vi "Sum of 3 Gaussians with offset fit.vi"() -> ()   [LabVIEW 2023]
doc: "Demonstrates fitting data to a model that is the sum of three Gaussian curves and an offset."
uses:
  <vilib>/Analysis/1siggen.llb/Ramp Pattern by Samples.vi
  <vilib>/gmath/NumericalOptimization/Nonlinear Curve Fit LM.vi
  <vilib>/gmath/NI_Gmath.lvlib
  <vilib>/Analysis/NI_AALBase.lvlib
  <vilib>/Analysis/NI_AAL_SigProc.lvlib
panel:
  out "Sum of 3 Gaussians":T1(graph)
  out "Number of function calls":i32
  out "Residue":dbl
  out "DC offset fit":dbl
  out "Gauss 3 fit":cluster{"a":dbl, "m":dbl, "sigma":dbl}
  out "Gauss 2 fit":cluster{"a":dbl, "m":dbl, "sigma":dbl}
  out "Gauss 1 fit":cluster{"a":dbl, "m":dbl, "sigma":dbl}
  in  "DC offset":dbl=4.0
  in  "Gauss 3":cluster{"a":dbl, "m":dbl, "sigma":dbl}={"a"=3.0, "m"=0.3, "sigma"=0.03}
  in  "Gauss 2":cluster{"a":dbl, "m":dbl, "sigma":dbl}={"a"=2.0, "m"=0.2, "sigma"=0.02}
  in  "Gauss 1":cluster{"a":dbl, "m":dbl, "sigma":dbl}={"a"=1.0, "m"=0.1, "sigma"=0.01}
  in  "Noise sigma":dbl(slide)=0.050505050505050504 scale=0.0..0.1
  # "Overview: Demonstrates fitting data to a model that is the sum of three Gaussian curves and an offset.\nRequirements: LabVIEW Full Development System\nInstructions:\n1.  Run the VI.\n2.  Notice the fit, which is mostly good.  Sometimes the smallest peak is missed due to the starting set of parameters for the fit.\n3.  Change the Gaussian parameters (DC offset, Gauss 1, Gauss 2, and Gauss 3) or Noise sigma and run the VI again."
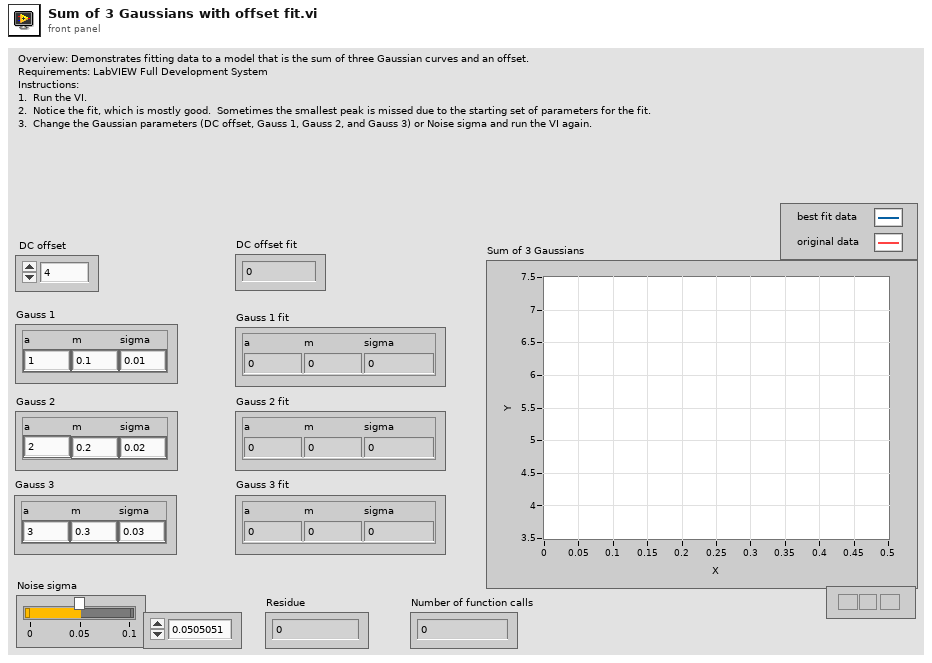
[diagram p1: front panel]
types:
  T1 = cluster{"Ramp Pattern":dbl[], "best nonlinear fit":dbl[]}[]
  T2 = cluster{"Ramp Pattern":dbl[], "best nonlinear fit":dbl[]}
  T3 = cluster{"Numeric":dbl, "Numeric":dbl, "Numeric":dbl}
  T4 = cluster{"Numeric":dbl, "Numeric":dbl, "Numeric":dbl}[]
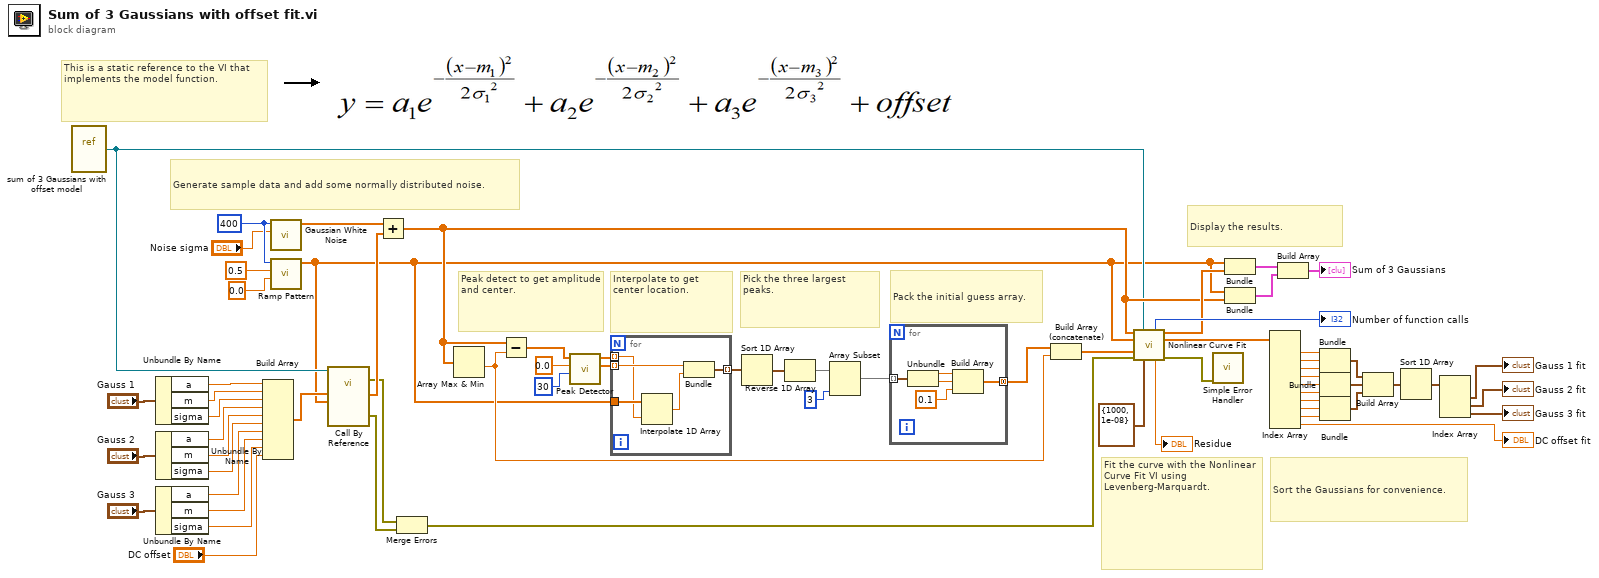
[diagram p0: block diagram]
diagram:
  w53 = 400 ("samples")
  # "Pack the initial guess array."
  # "Pick the three largest peaks."
  # "Peak detect to get amplitude and center."
  # "Sort the Gaussians for convenience."
  # "Generate sample data and add some normally distributed noise."
  # "Display the results."
  # "Fit the curve with the Nonlinear Curve Fit VI using Levenberg-Marquardt."
  # "Interpolate to get center location."
  # "This is a static reference to the VI that implements the model function."
  n1 = vi-ref "sum of 3 Gaussians with offset model.vi"() -> (w3:refnum<vi>)
  n2 = Unbundle By Name("Gauss 1") -> ("a"=w65:dbl, "m"=w64:dbl, "sigma"=w63:dbl)
  n3 = Unbundle By Name("Gauss 2") -> ("a"=w62:dbl, "m"=w61:dbl, "sigma"=w60:dbl)
  n4 = Unbundle By Name("Gauss 3") -> ("a"=w59:dbl, "m"=w58:dbl, "sigma"=w57:dbl)
  n5 = Build Array(w65, w64, w63, w62, w61, w60, w59, w58, w57, "DC offset") -> (w11:dbl[])
  n6 = call <vilib>:"Gaussian White Noise.vi"("standard deviation"="Noise sigma", "samples"=w53) -> ("Gaussian noise pattern"=w51:dbl[])  [unwired: 8 in, 1 out]
  n7 = call-poly <vilib>:"Ramp Pattern.vi"("start"=0.0, "end"=0.5, "samples"=w53) -> ("Ramp Pattern"=w2:dbl[])  [unwired: 7 in, 1 out]
  n8 = call-by-ref "?"(reference=w3, "X"=w2, "a"=w11) -> (error out=w6:errorcluster, 0:"error out"=w5:errorcluster, "f(X,a)"=w50:dbl[])  [unwired: 3 in, 2 out]
  n9 = Add(x=w51, y=w50) -> (x+y=w17:dbl[])
  n10 = Merge Errors(w6, w5) -> (w4:errorcluster)
  n11 = Array Max & Min(array=w17) -> (min value=w9:dbl)  [unwired: 3 out]
  n12 = Subtract(x=w17, y=w9) -> (x-y=w16:dbl[])
  n13 = call <vilib>:"Peak Detector.vi"("width"=30, "threshold"=0.0, "X"=w16) -> ("Amplitudes"=w20:dbl[], "Locations"=w19:dbl[])  [unwired: 4 in, 3 out]
  n14 = for {
    tunnel: w20 -> [w71] mode=indexing
    tunnel: w19 -> [w68] mode=indexing
    tunnel: [w70] -> w18 mode=indexing
    tunnel: w2 -> [w69]
    n15 = Interpolate 1D Array(1:w68, 2:w69) -> (0:w67:dbl)
    n16 = Bundle(w71, w67) -> (w70:cluster{dbl, dbl})  [unwired: 1 in]
  }
  n17 = Sort 1D Array(array=w18) -> (sorted array=w15:cluster{dbl, dbl}[])
  n18 = Reverse 1D Array(array=w15) -> (reversed array=w14:cluster{dbl, dbl}[])
  n19 = Array Subset(array=w14, length=3) -> (w10:cluster{dbl, dbl}[])  [unwired: 1 in]
  n20 = for {
    tunnel: w10 -> [w76] mode=indexing
    tunnel: [w72] -> w1 mode=concatenating
    n21 = Unbundle(w76) -> (w75:dbl, w74:dbl)
    n22 = Build Array(w75, w74, 0.1) -> (w72:dbl[])
  }
  n23 = Build Array (concatenate)(w1, w9) -> (w8:dbl[])
  n24 = call-poly <vilib>:"Nonlinear Curve Fit.vi"("Y"=w17, "f(x,a)"=w3, "X"=w2, "initial parameters"=w8, "error in (no error)"=w4, "termination"=cluster{"max iteration":i32, "tolerance":dbl} {"max iteration"=1000, "tolerance"=1e-08}) -> ("number of function calls"=→"Number of function calls":i32, "best nonlinear fit"=w49:dbl[], "best fit parameters"=w47:dbl[], "residue"=→"Residue":dbl, "error out"=w7:errorcluster)  [unwired: 4 in, 1 out]
  n25 = call <vilib>:"Simple Error Handler.vi"("error in (no error)"=w7) -> ()  [unwired: 4 in, 5 out]
  n26 = Bundle("Ramp Pattern"=w2, "best nonlinear fit"=w49) -> (w33:T2)  [unwired: 1 in]
  n27 = Bundle("Ramp Pattern"=w2, w17) -> (w34:cluster{"Ramp Pattern":dbl[], dbl[]})  [unwired: 1 in]
  n28 = Index Array(array=w47) -> (element #1=w46:dbl, element #2=w45:dbl, element #3=w44:dbl, element #4=w43:dbl, element #5=w42:dbl, element #6=w41:dbl, element #7=w40:dbl, element #8=w39:dbl, element #9=w38:dbl, element #10=→"DC offset fit":dbl)  [unwired: 10 in]
  n29 = Build Array(w33, w34) -> (→"Sum of 3 Gaussians":T1)
  n30 = Bundle("Numeric"=w46, "Numeric"=w45, "Numeric"=w44) -> (w29:T3)  [unwired: 1 in]
  n31 = Bundle("Numeric"=w43, "Numeric"=w42, "Numeric"=w41) -> (w28:T3)  [unwired: 1 in]
  n32 = Bundle("Numeric"=w40, "Numeric"=w39, "Numeric"=w38) -> (w27:T3)  [unwired: 1 in]
  n33 = Build Array(w29, w28, w27) -> (w26:T4)
  n34 = Sort 1D Array(array=w26) -> (sorted array=w25:T4)
  n35 = Index Array(array=w25) -> (element #1=→"Gauss 1 fit":T3, element #2=→"Gauss 2 fit":T3, element #3=→"Gauss 3 fit":T3)  [unwired: 3 in]
